vi "Level.vi"() -> ()   [LabVIEW 2011]
uses:
  Laba3/Global.vi
panel:
  in  "Стоп":bool
  in  "Пуск":bool
  out "Waveform Chart":dbl(graph)
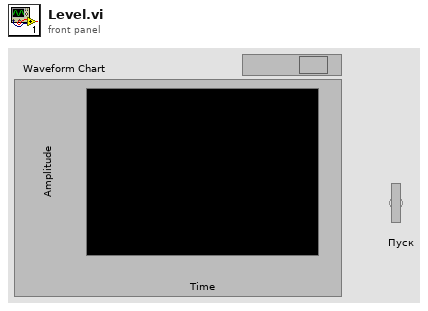
[diagram p1: front panel]
types:
  T1 = enum8{"Enabled", "Disabled", "Disabled and Grayed Out"}
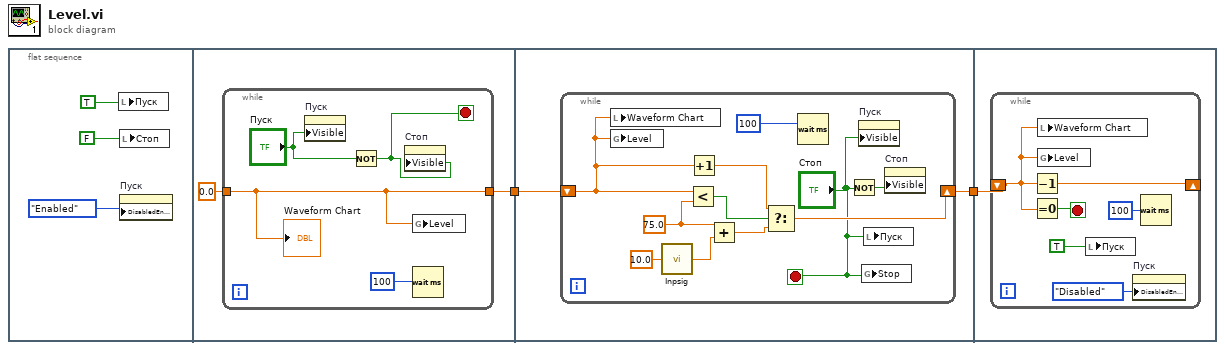
[diagram p0: block diagram]
diagram:
  n1 = flat-sequence {
    tunnel: [w7] -> w1
    tunnel: [w13] -> w2
    tunnel: w1 -> [w12]
    tunnel: w2 -> [w25]
    frame #0 {
      n2 = local write "Пуск"(TRUE) -> ()
      n3 = local write "Стоп"(FALSE ("Стоп")) -> ()
      n4 = property on="Пуск" class="Bool (strict)"("DisabledEnum"=T1."Enabled" ("Disabled")) -> ()  [unwired: 2 in, 2 out]
    }
    frame #1 {
      n5 = while {
        tunnel: [w8] -> w7
        tunnel: 0.0 -> [w8]
        stop <- w10 stop-if-true
        n6 = property on="Пуск" class="Bool (strict)"("Visible"="Пуск") -> ()  [unwired: 2 in, 2 out]
        n7 = Not(x="Пуск") -> (.not. x?=w10:bool)
        n8 = property on="Стоп" class="Bool (strict)"("Visible"=w10) -> ()  [unwired: 2 in, 2 out]
        n9 = global write "Global.vi" "Level"(w8) -> ()
        n10 = Wait (ms)(milliseconds to wait=100) -> ()  [unwired: 1 out]
        "Waveform Chart" <- w8
      }
    }
    frame #2 {
      n11 = while {
        shift-right: [w21] -> w13
        shift-left: w12 -> [w19]
        stop <- "Стоп" stop-if-true
        w22 = 75.0
        n12 = local write "Waveform Chart"(w19) -> ()
        n13 = global write "Global.vi" "Level"(w19) -> ()
        n14 = call "Inpsig.vi"("Множитель"=10.0) -> ("Случайное число"=w16:dbl)
        n15 = Less?(x=w19, y=w22) -> (x < y?=w18:bool)
        n16 = Increment(x=w19) -> (x+1=w23:dbl)
        n17 = Add(x=w22, y=w16) -> (x+y=w24:dbl)
        n18 = Select(t=w23, s=w18, f=w24) -> (s? t:f=w21:dbl)
        n19 = Wait (ms)(milliseconds to wait=100) -> ()  [unwired: 1 out]
        n20 = Not(x="Стоп") -> (.not. x?=w17:bool)
        n21 = property on="Пуск" class="Bool (strict)"("Visible"="Стоп") -> ()  [unwired: 2 in, 2 out]
        n22 = global write "Global.vi" "Stop"("Стоп") -> ()
        n23 = local write "Пуск"("Стоп") -> ()
        n24 = property on="Стоп" class="Bool (strict)"("Visible"=w17) -> ()  [unwired: 2 in, 2 out]
      }
    }
    frame #3 {
      n25 = while {
        shift-right: [w29] -> _
        shift-left: w25 -> [w28]
        stop <- w31 stop-if-true
        n26 = Decrement(x=w28) -> (x-1=w29:dbl)
        n27 = Equal To 0?(x=w28) -> (x = 0?=w31:bool)
        n28 = local write "Waveform Chart"(w28) -> ()
        n29 = global write "Global.vi" "Level"(w28) -> ()
        n30 = local write "Пуск"(TRUE) -> ()
        n31 = property on="Пуск" class="Bool (strict)"("DisabledEnum"=T1."Disabled" ("Disabled")) -> ()  [unwired: 2 in, 2 out]
        n32 = Wait (ms)(milliseconds to wait=100) -> ()  [unwired: 1 out]
      }
    }
  }
